vi "run.vi"(8 "error in (no error)":errorcluster, 11 "Protocol_MoveToSetpoint in":refnum<class "Protocol_MoveToSetpoint.lvclass">) -> (0 "error out":errorcluster, 3 "Protocol_MoveToSetpoint out":refnum<class "Protocol_MoveToSetpoint.lvclass">)   [LabVIEW 2011, in "Protocol_MoveToSetpoint.lvclass"]
uses:
  Protocol_MoveToSetpoint.lvclass
  protocol_Generic/Protocol_Generic.lvclass
  Protocol_MoveToSetpoint.lvclass/Protocol_MoveToSetpoint.ctl
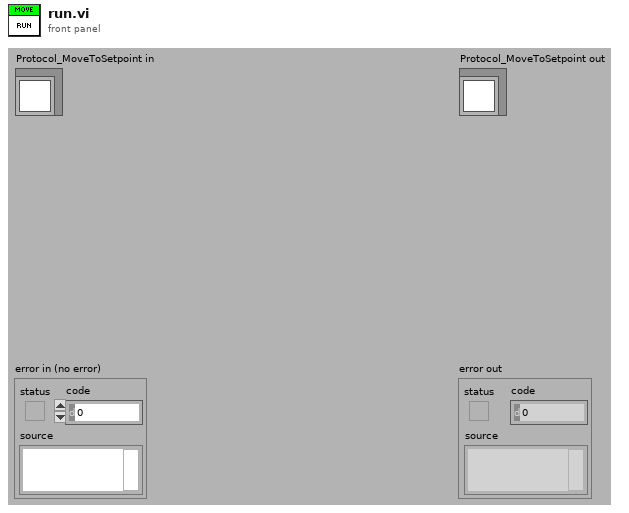
[diagram p1: front panel]
types:
  T1 = cluster{"Axis Information":cluster{"Device ID":i32, "Device Name":string, "Device Type":i32}[], "Axis Selector":i32[], "Control Modes out":u16[], "error out":errorcluster, "Channel Data":cluster{"Name":string, "Type":i32, "SI Full Scale":dbl, "Full Scale":dbl, "Units String":string, "Display Format":string, "Gauge Length":dbl}[][]}
  T2 = cluster{"Device ID":i32, "Device Name":string, "Device Type":i32}[]
  T3 = cluster{"Name":string, "Type":i32, "SI Full Scale":dbl, "Full Scale":dbl, "Units String":string, "Display Format":string, "Gauge Length":dbl}[][]
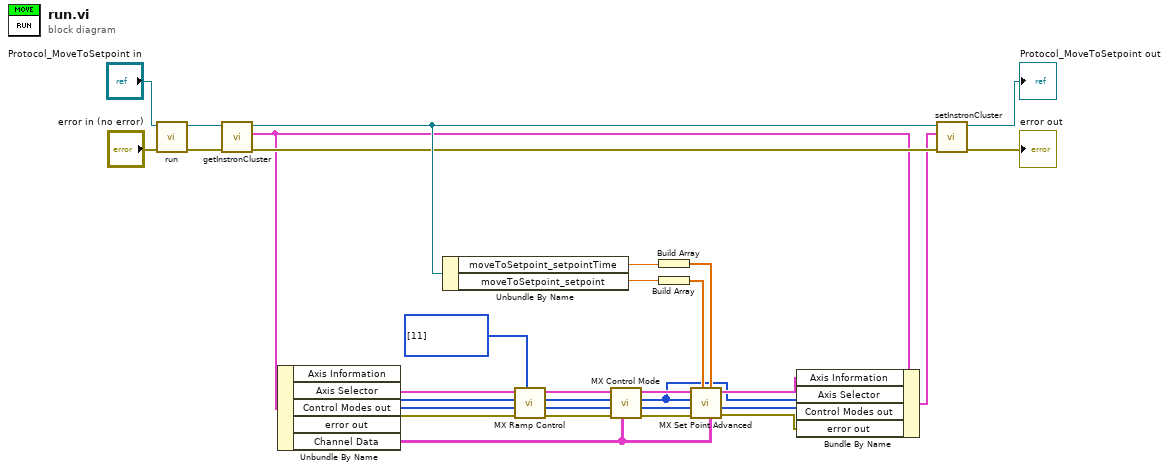
[diagram p0: block diagram]
diagram:
  w19 = u16[] [11] items=["Stop", "Start or continue", "Hold", "Continue", "Return ramp to set level at fixed rate", "Reserved", "Reserved", "Start Random without demand hold", "Start Random with demand hold", "Prepare Random Start without demand hold", "Prepare Random Start with demand hold", "Unslave", "Reserved", "Reserved", "Start Sample Data Playback or Resume", "Prepare for Start of Sample Data", "Reserved", "Reserved", "Resume Playback", "Start an electromechanical frame return"] ("Ramp Control")
  n1 = call-parent "run.vi"("error in (no error)"="error in (no error)", "Protocol_Generic in"="Protocol_MoveToSetpoint in") -> ("error out"=w8:errorcluster, "Protocol_Generic out"=w31:refnum<class "Protocol_MoveToSetpoint.lvclass">)  [unwired: 8 in]
  n2 = call-dynamic "getInstronCluster.vi"("error in (no error)"=w8, "Protocol_Generic in"=w31) -> ("error out"=w4:errorcluster, "InstronCluster"=w1:T1, "Protocol_Generic out"=w6:refnum<class "Protocol_MoveToSetpoint.lvclass">)  [unwired: 7 in]
  n3 = Unbundle By Name(w1) -> ("Axis Information"=w16:T2, "Axis Selector"=w15:i32[], "Control Modes out"=w7:u16[], "error out"=w14:errorcluster, "Channel Data"=w13:T3)
  n4 = Unbundle By Name(w6) -> ("moveToSetpoint_setpointTime"=w18:dbl, "moveToSetpoint_setpoint"=w17:dbl)
  n5 = call "MX Ramp Control.vi"("Ramp Control"=w19, "error in (no error)"=w14, "Channels In"=w7, "Axis Selector In"=w15, "Axis Information In"=w16) -> ("error out"=w22:errorcluster, "Channels Out"=w23:u16[], "Axis Selector Out"=w24:i32[], "Axis Information Out"=w25:T2)  [unwired: 2 in]
  n6 = call "MX Control Mode.vi"("Channel Data"=w13, "error in (no error)"=w22, "Control Modes"=w23, "Axis Selector"=w24, "Axis Information"=w25) -> ("error out"=w28:errorcluster, "Control Modes out"=w26:u16[], "Axis Selector out"=w11:i32[], "Axis Information out"=w27:T2)  [unwired: 1 in]
  n7 = Build Array(w18) -> (w20:dbl[])
  n8 = Build Array(w17) -> (w21:dbl[])
  n9 = call "MX Set Point Advanced.vi"("Channel Data"=w13, "Time"=w20, "Set Point"=w21, "error in (no error)"=w28, "Channels"=w26, "Axis Selector"=w11, "Axis Information"=w27) -> ("error out"=w9:errorcluster, "Channels out"=w10:u16[], "Axis Information out"=w12:T2)  [unwired: 2 in]
  n10 = Bundle By Name(cluster=w1, "Axis Information"=w12, "Axis Selector"=w11, "Control Modes out"=w10, "error out"=w9) -> (w2:T1)
  n11 = call-dynamic "setInstronCluster.vi"("error in (no error)"=w4, "InstronCluster"=w2, "Protocol_Generic in"=w6) -> ("error out"=→"error out":errorcluster, "Protocol_Generic out"=→"Protocol_MoveToSetpoint out":refnum<class "Protocol_MoveToSetpoint.lvclass">)  [unwired: 7 in]
